vi "Climb_Solenoid.vi"(8 "Left Bottom Right":bool, 9 "Left Bottom Left":bool, 10 "Left Top Left":bool, 11 "Left Top Right":bool) -> ()   [LabVIEW 2020]
uses:
  <vilib>/Rock Robotics/WPI/Solenoid/WPI_SolenoidSetEnum.vi
  <vilib>/Rock Robotics/WPI/Solenoid/WPI_SolenoidValue.ctl
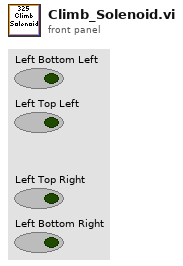
[diagram p1: front panel]
types:
  T1 = typedef "WPI_SolenoidDevRef.ctl" = cluster{"DevStatus":errorcluster, "Pneumatics Control Module":u8, "Forward Solenoid Channel":T2, "Reverse Solenoid Channel":T2}
  T2 = typedef "WPI_SolenoidChannel.ctl" = enum8{"Solenoid 0", "Solenoid 1", "Solenoid 2", "Solenoid 3", "Solenoid 4", "Solenoid 5", "Solenoid 6", "Solenoid 7", "Solenoid 8", "Solenoid 9", "Solenoid 10", "Solenoid 11", "Solenoid 12", "Solenoid 13", "Solenoid 14", "Solenoid 15", "Invalid"}
  T3 = typedef "WPI_SolenoidValue.ctl" = enum16{"Off", "On", "Forward", "Reverse"}
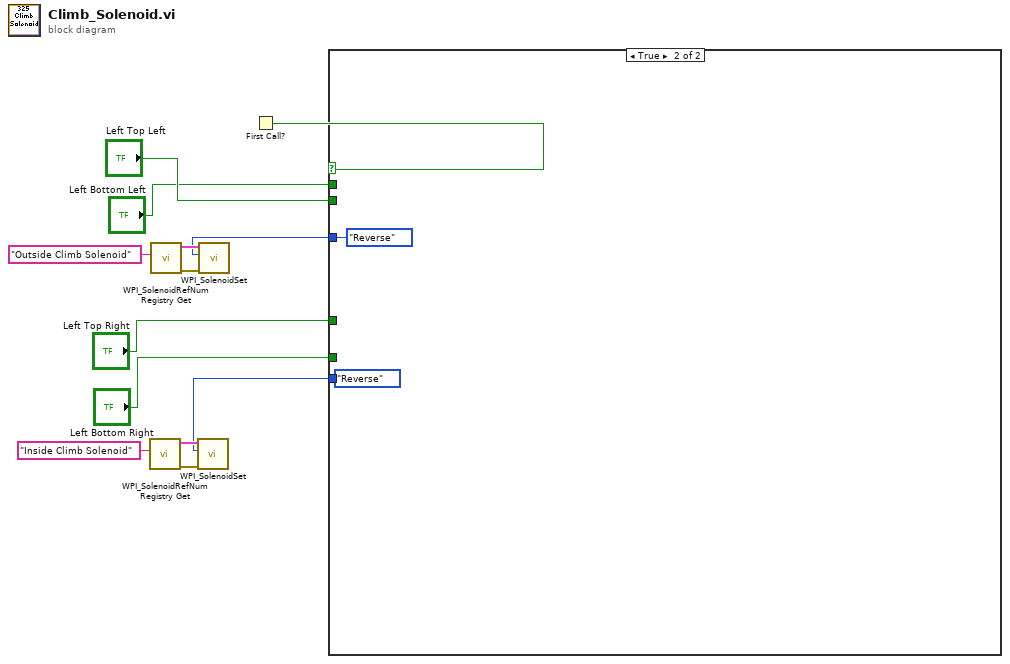
[diagram p0: block diagram]
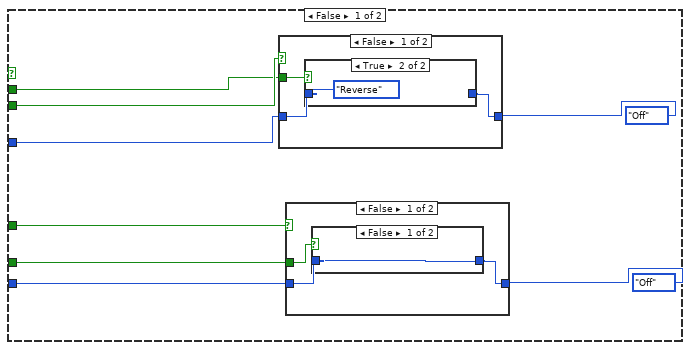
[diagram p2: hidden frame]
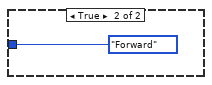
[diagram p4: hidden frame]
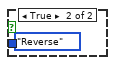
[diagram p5: hidden frame]
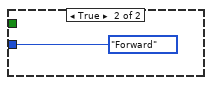
[diagram p6: hidden frame]
diagram:
  n1 = call <vilib>:"WPI_SolenoidRefNum Registry Get.vi"("refnum name"="Inside Climb Solenoid") -> ("error out"=w12:errorcluster, "SolenoidDevRef"=w11:T1)  [unwired: 9 in]
  n2 = call <vilib>:"WPI_SolenoidRefNum Registry Get.vi"("refnum name"="Outside Climb Solenoid") -> ("error out"=w6:errorcluster, "SolenoidDevRef"=w5:T1)  [unwired: 9 in]
  n3 = First Call?() -> (First Call?: T/F=w13:bool)
  n4 = case shown="True" w13 {
    tunnel: [w19 WPI_SolenoidValue."Reverse" ("inside climb start")] -> w10
    tunnel: "Left Bottom Right" -> [w18 _]
    tunnel: "Left Top Right" -> [w17 _]
    tunnel: [w16 WPI_SolenoidValue."Reverse" ("inside climb start")] -> w4
    tunnel: "Left Top Left" -> [w15 _]
    tunnel: "Left Bottom Left" -> [w14 _]
    frame False {
      n5 = case shown="False" w15 {
        tunnel: [w23 WPI_SolenoidValue."Forward" ("inside climb start")] -> w16
        tunnel: WPI_SolenoidValue."Off" ("inside climb start") -> [w24 _]
        tunnel: w14 -> [w22 _]
        frame False {
          n6 = case shown="True" w22 {
            tunnel: w24 -> [w25 _]
            tunnel: [w25 WPI_SolenoidValue."Reverse" ("inside climb start")] -> w23
            frame False {
            }
            frame True {
            }
          }
        }
        frame True {
        }
      }
      n7 = case shown="False" w17 {
        tunnel: [w29 WPI_SolenoidValue."Forward" ("inside climb start")] -> w19
        tunnel: WPI_SolenoidValue."Off" ("inside climb start") -> [w30 _]
        tunnel: w18 -> [w28 _]
        frame False {
          n8 = case shown="False" w28 {
            tunnel: w30 -> [w31 _]
            tunnel: [w31 WPI_SolenoidValue."Reverse" ("inside climb start")] -> w29
            frame False {
            }
            frame True {
            }
          }
        }
        frame True {
        }
      }
    }
    frame True {
    }
  }
  n9 = call-poly <vilib>:"WPI_SolenoidSet.vi"("error in (no error)"=w12, "Value"=w10, "SolenoidDevRef"=w11) -> ()  [unwired: 7 in, 2 out]
  n10 = call-poly <vilib>:"WPI_SolenoidSet.vi"("error in (no error)"=w6, "Value"=w4, "SolenoidDevRef"=w5) -> ()  [unwired: 7 in, 2 out]
